vi "distance calculation.vi"(1 "Antenna  position (ECI coordinates)":T1, 2 "Satellite position (ECI coordinates)":T1) -> (0 "Distance (km)":dbl)   [LabVIEW 2015]
uses:
  <vilib>/Analysis/Matrix/Datatypes/RealMatrix.ctl
  <vilib>/Analysis/Matrix/NI_Matrix.lvlib
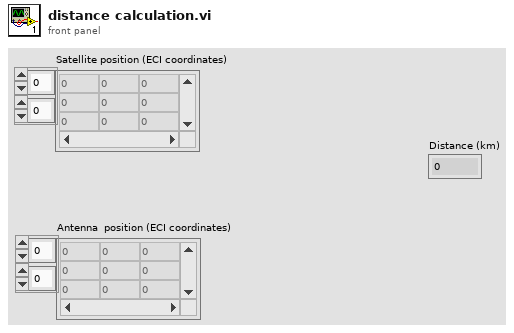
[diagram p1: front panel]
types:
  T1 = typedef "NI_Matrix.lvlib/RealMatrix.ctl" = dbl[][]
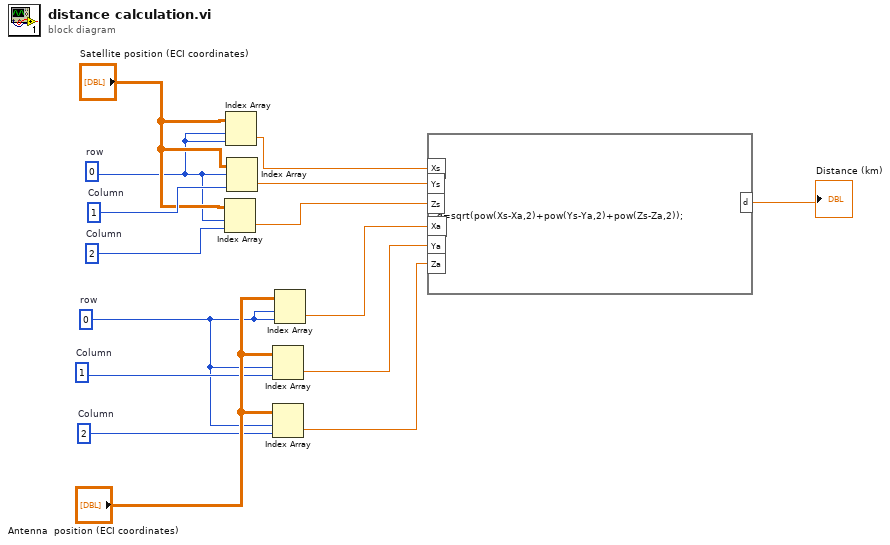
[diagram p0: block diagram]
diagram:
  w6 = 2  # Column
  w7 = 1  # Column
  w5 = 0  # row
  w9 = 2  # Column
  w13 = 1  # Column
  w10 = 0  # row
  n1 = Index Array(array="Satellite position (ECI coordinates)", index (row)=w10, index (col)=w9) -> (element=w14:dbl)
  n2 = Index Array(array="Satellite position (ECI coordinates)", index (row)=w10, index (col)=w10) -> (element=w15:dbl)
  n3 = Index Array(array="Satellite position (ECI coordinates)", index (row)=w10, index (col)=w13) -> (element=w12:dbl)
  n4 = Index Array(array="Antenna  position (ECI coordinates)", index (row)=w5, index (col)=w7) -> (element=w3:dbl)
  n5 = Index Array(array="Antenna  position (ECI coordinates)", index (row)=w5, index (col)=w6) -> (element=w2:dbl)
  n6 = Index Array(array="Antenna  position (ECI coordinates)", index (row)=w5, index (col)=w5) -> (element=w4:dbl)
  n7 = formula code="d=sqrt(pow(Xs-Xa,2)+pow(Ys-Ya,2)+pow(Zs-Za,2));"("Xs"=w15, "Ys"=w12, "Zs"=w14, "Xa"=w4, "Ya"=w3, "Za"=w2) -> ("d"=→"Distance (km)":dbl)
